vi "tb_Input Multiplexer(4 Inputs)_host.vi"() -> ()   [LabVIEW 2010]
uses:
  Input Index(Type) 4 inputs.ctl
panel:
  in  "Reset?":bool
  out "transposed array":T1[][](array[typedef])
  out "Numeric":i32
  out "appended array":bool[][](array[boolean])
  out "MIndex3":T1
  out "MIndex2":T1
  out "MIndex1":T1
  out "MIndex0":T1
  out "Data Valid":bool[](array[boolean])
  out "Sorted Data":i16[](array[numeric])
  in  "Data Valid":bool[](array[boolean])=[FALSE, FALSE, FALSE, FALSE]
  in  "Data":i16[](array[numeric])=[0, 0, 0, 0]
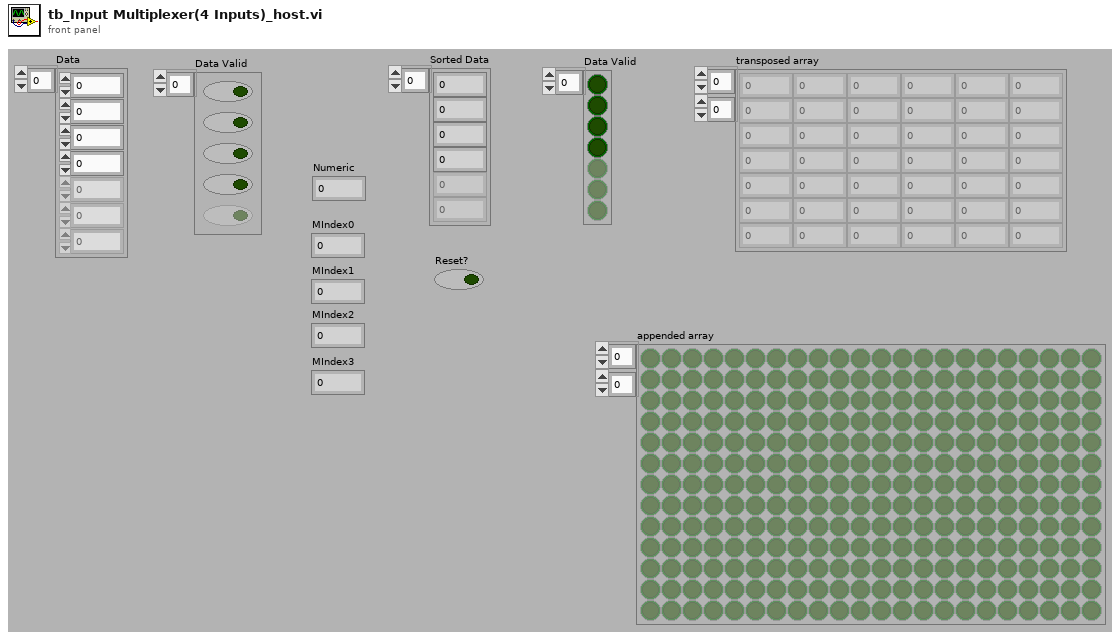
[diagram p1: front panel]
types:
  T1 = typedef "Input Index(Type) 4 inputs.ctl" = fxp<+,2,2>
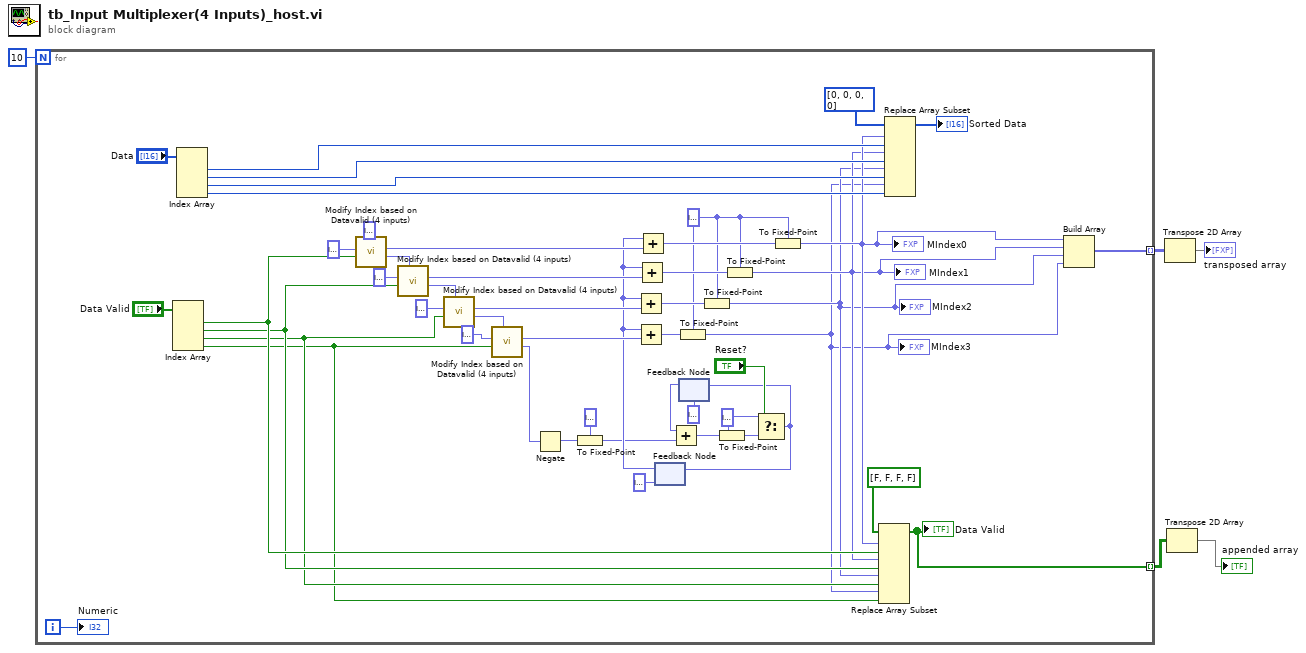
[diagram p0: block diagram]
diagram:
  n1 = for {
    N: 10 -> [_]
    tunnel: [w19] -> w4 mode=indexing
    tunnel: [w13] -> w2 mode=indexing
    i -> [w18]
    w20 = T1 0.0
    w8 = T1 0.0 ("Actual Index")
    n2 = Index Array(array="Data Valid") -> (element #1=w46:bool, element #2=w45:bool, element #3=w44:bool, element #4=w43:bool)  [unwired: 4 in]
    n3 = Index Array(array="Data") -> (element #1=w33:i16, element #2=w32:i16, element #3=w31:i16, element #4=w30:i16)  [unwired: 4 in]
    n4 = call "Modify Index based on Datavalid (4 inputs).vi"("previous counter val"=T1 0.0, "cuurent index data valid?"=w46, "Actual Index"=T1 0.0) -> ("Next Counter Val"=w49:T1, "Modified Index"=w42:T1)  [unwired: 7 in]
    n5 = call "Modify Index based on Datavalid (4 inputs).vi"("previous counter val"=w49, "cuurent index data valid?"=w45, "Actual Index"=T1 1.0) -> ("Next Counter Val"=w48:T1, "Modified Index"=w40:T1)  [unwired: 7 in]
    n6 = call "Modify Index based on Datavalid (4 inputs).vi"("previous counter val"=w48, "cuurent index data valid?"=w44, "Actual Index"=T1 2.0) -> ("Next Counter Val"=w47:T1, "Modified Index"=w39:T1)  [unwired: 7 in]
    n7 = call "Modify Index based on Datavalid (4 inputs).vi"("previous counter val"=w47, "cuurent index data valid?"=w43, "Actual Index"=T1 3.0) -> ("Next Counter Val"=w22:T1, "Modified Index"=w38:T1)  [unwired: 7 in]
    n8 = Negate(x=w22) -> (-x=w12:fxp<+/-,3,3>)
    n9 = To Fixed-Point(fixed-point type=T1 0.0 ("Current Index Sum"), number=w12) -> (fixed-point=w11:T1)
    n10 = feedback #1(T1 0.0 ("Current Index Sum")) -> (w36:T1)
    n11 = Add(x=w36, y=w39) -> (x+y=w24:fxp<+,3,3>)
    n12 = Add(x=w36, y=w38) -> (x+y=w23:fxp<+,3,3>)
    n13 = Add(x=w36, y=w40) -> (x+y=w25:fxp<+,3,3>)
    n14 = Add(x=w36, y=w42) -> (x+y=w41:fxp<+,3,3>)
    n15 = To Fixed-Point(fixed-point type=w20, number=w23) -> (fixed-point=w14:T1)
    "MIndex3" <- w14
    n16 = feedback #2(T1 0.0) -> (w35:T1)
    n17 = Add(x=w35, y=w11) -> (x+y=w21:fxp<+,3,3>)
    n18 = To Fixed-Point(fixed-point type=w20, number=w24) -> (fixed-point=w15:T1)
    "MIndex2" <- w15
    n19 = To Fixed-Point(fixed-point type=w8, number=w21) -> (fixed-point=w9:T1)
    n20 = To Fixed-Point(fixed-point type=w20, number=w25) -> (fixed-point=w16:T1)
    "MIndex1" <- w16
    n21 = Select(t=w8, s="Reset?", f=w9) -> (s? t:f=w6:T1)
    n22 = feedback-in #1(w6) -> ()
    n23 = feedback-in #2(w6) -> ()
    n24 = To Fixed-Point(fixed-point type=w20, number=w41) -> (fixed-point=w17:T1)
    "MIndex0" <- w17
    n25 = Replace Array Subset(array=bool[] [FALSE, FALSE, FALSE, FALSE] ("appended array"), new element #1=w46, index #1=w17, new element #2=w45, index #2=w16, new element #3=w44, index #3=w15, new element #4=w43, index #4=w14) -> (w19:bool[])
    "Data Valid" <- w19
    n26 = Replace Array Subset(array=i16[] [0, 0, 0, 0], new element #1=w33, index #1=w17, new element #2=w32, index #2=w16, new element #3=w31, index #3=w15, new element #4=w30, index #4=w14) -> (→"Sorted Data":i16[])
    n27 = Build Array(w17, w16, w15, w14) -> (w13:T1[])
    "Numeric" <- w18
  }
  n28 = Transpose 2D Array(2D array=w2) -> (transposed array=→"transposed array":T1[][])
  n29 = Transpose 2D Array(2D array=w4) -> (transposed array=→"appended array":bool[][])
